vi "TEMOCR-Restore Defaults.vi"() -> (8 "Params":T1={"Probe"={"Ear"=enum."Right", "Stimulus"=enum."Click", "Duration (us)"=100.0, "Nclick"=4, "ICI (ms)"=32.0, "Level"=65.0}, "Elicitor"={"Onset (s)"=2.0, "Offset (s)"=10.0, "Ramp (ms)"=2.5, "Transducer"=enum."Insert"}, "Sequence"={"Start"=40.0, "Stop"=92.0, "Step"=4.0}, "Analysis"={"Tmin (ms)"=2.0, "Tmax (ms)"=16.0, "Fmin (Hz)"=800.0, "Fmax (Hz)"=3200.0, "Window"=enum."Hamming", "Fhp (Hz)"=750.0, "Flp (Hz)"=5000.0, "Gain (dB)"=40.0}, "Repeats"=500, "Fs (Hz)"=50000.0, "Cycles"=1, "save raw"=FALSE})   [LabVIEW 2015]
uses:
  Typedefs/TEMOCR-Parameters.ctl
  Typedefs/TEMOCR-Probe.ctl
  Typedefs/TEMOCR-Elicitor.ctl
  Human Studies/SFM Frontend/LV Source/Typedefs/HSTS-Transducer.ctl
  Typedefs/TEMOCR-Sequence.ctl
  Typedefs/TEMOCR-Analysis.ctl
panel:
  out "error out":errorcluster
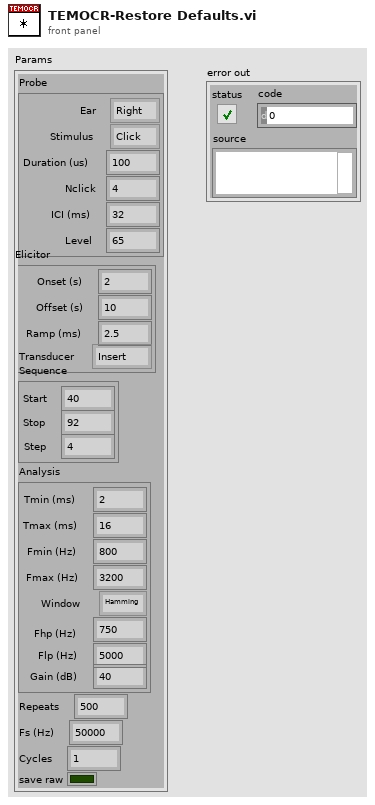
[diagram p1: front panel]
types:
  T1 = typedef "TEMOCR-Parameters.ctl" = cluster{"Probe":T2, "Elicitor":T3, "Sequence":T5, "Analysis":T6, "Repeats":i32, "Fs (Hz)":dbl, "Cycles":i32, "save raw":bool}
  T2 = typedef "TEMOCR-Probe.ctl" = cluster{"Ear":enum16{"Right", "Left"}, "Stimulus":enum16{"Click", "Chirp"}, "Duration (us)":dbl, "Nclick":i32, "ICI (ms)":dbl, "Level":dbl}
  T3 = typedef "TEMOCR-Elicitor.ctl" = cluster{"Onset (s)":dbl, "Offset (s)":dbl, "Ramp (ms)":dbl, "Transducer":T4}
  T4 = typedef "HSTS-Transducer.ctl" = enum16{"Insert", "TDH-39", "HD300", "ER-10X"}
  T5 = typedef "TEMOCR-Sequence.ctl" = cluster{"Start":dbl, "Stop":dbl, "Step":dbl}
  T6 = typedef "TEMOCR-Analysis.ctl" = cluster{"Tmin (ms)":dbl, "Tmax (ms)":dbl, "Fmin (Hz)":dbl, "Fmax (Hz)":dbl, "Window":enum16{"None", "Hanning", "Hamming"}, "Fhp (Hz)":dbl, "Flp (Hz)":dbl, "Gain (dB)":dbl}
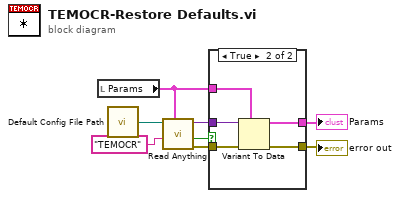
[diagram p0: block diagram]
diagram:
  n1 = local read "Params"() -> (w3:T1)
  n2 = call "Default Config File Path.vi"() -> ("Default config file name"=w8:path)
  n3 = call "Read Anything.vi"("Type of Anything"=w3, "Section Name (Name of \"Type of Anything\")"="TEMOCR" ("Section Name (Name of \"Type of Anything\")"), "Path (dialog)"=w8) -> ("Error Out"=w5:errorcluster, "Found?"=w4:bool, "Anything"=w6:variant)  [unwired: 6 in]
  n4 = case shown="True" w4 {
    tunnel: w6 -> [_ w14]
    tunnel: w5 -> [w9 w15]
    tunnel: w3 -> [w10 w13]
    tunnel: [w10 w12] -> w2
    tunnel: [w9 w11] -> w1
    frame False {
    }
    frame True {
      n5 = Variant To Data(error in=w15, type=w13, Variant=w14) -> (data=w12:T1, error out=w11:errorcluster)
    }
  }
  "Params" <- w2
  "error out" <- w1
